vi "MB ICPCON Registers Read DOs.vi"(7 "Data Reference":T1, 8 "error in (no error)":errorcluster, 10 "Length":i32, 11 "N":i32) -> (0 "error out":errorcluster, 1 "Bits out":bool[][](array[boolean]))   [LabVIEW 2019, in "ICPCON Registers.lvlib"]
uses:
  ICPCON Registers.lvlib
  Ctl/ICPCON Data.ctl
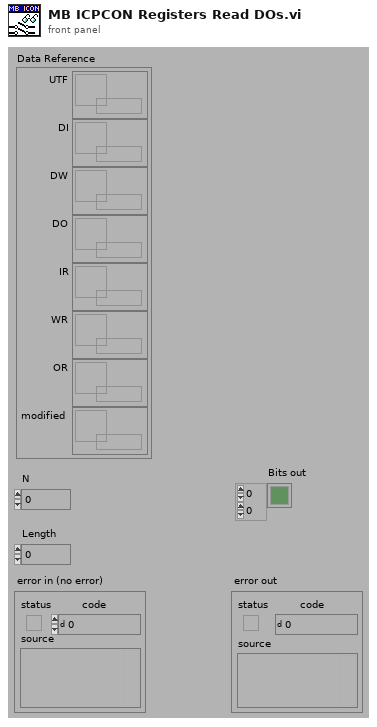
[diagram p1: front panel]
types:
  T1 = typedef "ICPCON Registers.lvlib/ICPCON Data.ctl" = cluster{"UTF":refnum<data-value>, "DI":refnum<data-value>, "DW":refnum<data-value>, "DO":refnum<data-value>, "IR":refnum<data-value>, "WR":refnum<data-value>, "OR":refnum<data-value>, "modified":refnum<data-value>}
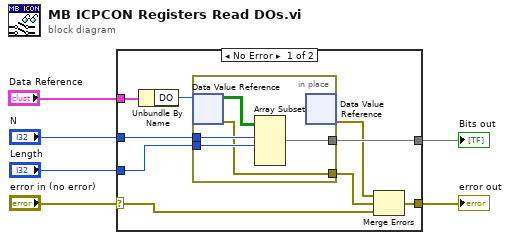
[diagram p0: block diagram]
diagram:
  n1 = case shown="No Error" "error in (no error)" {
    selector: "error in (no error)" -> [w7 w21]
    tunnel: [w11 w21] -> w6
    tunnel: [w15 _] -> w5
    tunnel: "Length" -> [w14 _]
    tunnel: "N" -> [w13 _]
    tunnel: "Data Reference" -> [w12 _]
    frame No Error {
      n2 = Unbundle By Name(w12) -> ("DO"=w8:refnum<data-value>)
      n3 = in-place {
        in-place-border: w13 -> [w20]
        in-place-border: w14 -> [w19]
        in-place-border: [w16] -> w15
        in-place-border: [w17] -> w9
        n4 = in-place-dvr #1(w8) -> (w18:bool[][], w17:errorcluster)
        n5 = Array Subset(array=w18, index (row)=w20, length (row)=w19) -> (w16:bool[][])  [unwired: 2 in]
        n6 = in-place-dvr #1() -> (w10:errorcluster)  [unwired: 1 in, 1 out]
      }
      n7 = Merge Errors(w10, w9, w7) -> (w11:errorcluster)
    }
    frame Error {
    }
  }
  "error out" <- w6
  "Bits out" <- w5
